vi "unpack_pose.vi"(11 "pose":u64) -> (2 "error":bool, 3 "pose":sgl[][](array[numeric]))   [LabVIEW 2023]
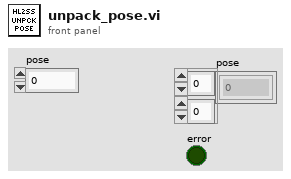
[diagram p1: front panel]
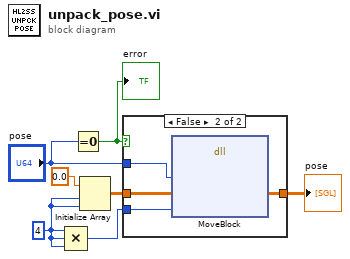
[diagram p0: block diagram]
diagram:
  w5 = 4 ("dimension size")
  n1 = Compound Arithmetic op=MULTIPLY(w5, w5, w5) -> (w4:i32)
  n2 = Equal To 0?(x="pose") -> (x = 0?=w2:bool)
  "error" <- w2
  n3 = Initialize Array(sgl 0.0 ("element"), w5, w5) -> (w6:sgl[][])
  n4 = case shown="False" w2 {
    tunnel: w6 -> [w8 w12]
    tunnel: w4 -> [_ w11]
    tunnel: "pose" -> [_ w10]
    tunnel: [w8 w9] -> w3
    frame True {
    }
    frame False {
      n5 = dll-call lib="LabVIEW" fn="MoveBlock"("ps"=w10, "pd"=w12, "size"=w11) -> ("pd"=w9:sgl[][])  [unwired: 6 in, 2 out]
    }
  }
  "pose" <- w3
